vi "JsonFile Save.vi"(8 "error in (no error)":errorcluster, 10 "JSON String":string, 11 "Path":path) -> (0 "error out":errorcluster)   [LabVIEW 2019, in "lv-apt-json-file.lvlib"]
uses:
  lv-apt-json-file.lvlib
  <vilib>/Utility/error.llb/Clear Errors.vi
  Json/Remove Comments.vi
  <userlib>/NEVSTOP-Programming-Palette/Configuration/Ini/TextToLines.vi
  <userlib>/_OpenG.lib/array/array.llb/Filter 1D Array__ogtk.vi
  <userlib>/_OpenG.lib/array/array.llb/Filter 1D Array (U8)__ogtk.vi
  <userlib>/NEVSTOP-Programming-Palette/Configuration/Ini/LinesToText.vi
  <vilib>/addons/_JKI.lib/Serialization/JSON/Library/Unflatten From JSON String.vi
  <vilib>/Utility/error.llb/Error Cluster From Error Code.vi
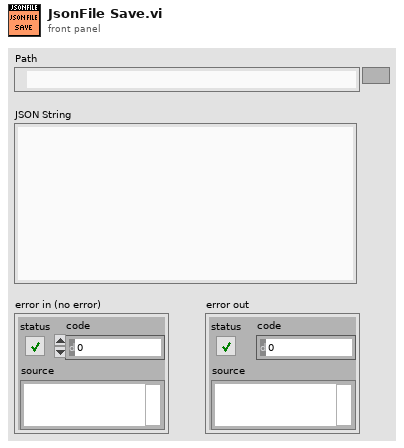
[diagram p1: front panel]
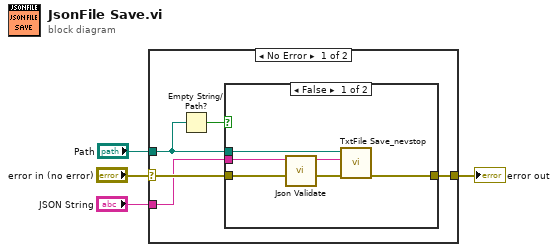
[diagram p0: block diagram]
diagram:
  n1 = case shown="No Error" "error in (no error)" {
    selector: "error in (no error)" -> [w7 w17]
    tunnel: [w9 w17] -> w4
    tunnel: "Path" -> [w6 _]
    tunnel: "JSON String" -> [w5 _]
    frame No Error {
      n2 = Empty String/Path?(string/path=w6) -> (empty?=w8:bool)
      n3 = case shown="False" w8 {
        tunnel: w7 -> [w11 w16]
        tunnel: [w15 w16] -> w9
        tunnel: w5 -> [w13 _]
        tunnel: w6 -> [w14 _]
        frame False {
          n4 = call "Json Validate.vi"("error in (no error)"=w11, "String"=w13) -> ("error out"=w10:errorcluster, "Json without comments"=w12:string)  [unwired: 6 in, 2 out]
          n5 = call <userlib>:"TxtFile Save_nevstop.vi"("error in (no error)"=w10, "text"=w12, "Path"=w14) -> ("error out"=w15:errorcluster)  [unwired: 8 in]
        }
        frame True {
        }
      }
    }
    frame Error {
    }
  }
  "error out" <- w4
